vi "Ensure Channel.vi"(8 "error in (no error)":errorcluster, 10 "Name":string, 11 "SignalManager in":refnum<class "SignalManager.lvclass">) -> (0 "error out":errorcluster, 3 "SignalManager out":refnum<class "SignalManager.lvclass">)   [LabVIEW 2015, in "SignalManager.lvclass"]
uses:
  SignalManager.lvclass
  SignalManager.lvclass/SignalManager.ctl
  Channel/Channel.lvclass
  Channel/Channel.lvclass/Channel.ctl
  Channel/Write Name.vi
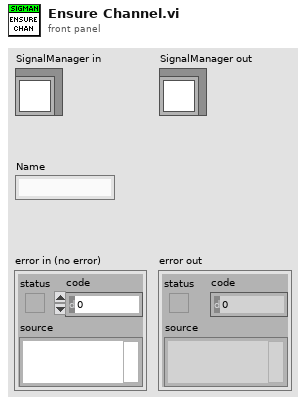
[diagram p1: front panel]
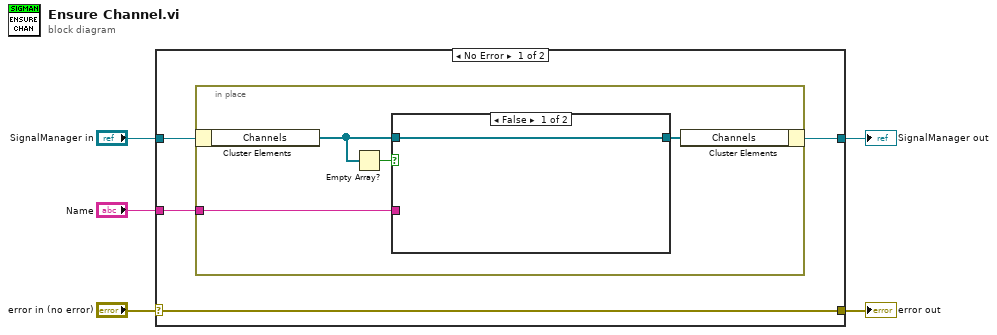
[diagram p0: block diagram]
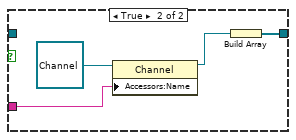
[diagram p2: hidden frame]
diagram:
  n1 = case shown="No Error" "error in (no error)" {
    selector: "error in (no error)" -> [w9 w20]
    tunnel: [w9 w20] -> w4
    tunnel: [w7 w19] -> w2
    tunnel: "SignalManager in" -> [w8 w19]
    tunnel: "Name" -> [w6 _]
    frame No Error {
      n2 = in-place {
        in-place-border: w6 -> [w10]
        n3 = in-place-cluster #1(w8) -> ("Channels"=w11:refnum<class "Channel.lvclass">[])
        n4 = Empty Array?(array=w11) -> (empty?=w12:bool)
        n5 = case shown="False" w12 {
          tunnel: [w14 w18] -> w13
          tunnel: w11 -> [w14 _]
          tunnel: w10 -> [_ w15]
          frame False {
          }
          frame True {
            n6 = property class="Channel"(reference=refnum<class "Channel.lvclass"> refnum ("Channel"), "Accessors:Name"=w15) -> (reference out=w16:refnum<class "Channel.lvclass">)  [unwired: 1 in, 1 out]
            n7 = Build Array(w16) -> (w18:refnum<class "Channel.lvclass">[])
          }
        }
        n8 = in-place-cluster #1("Channels"=w13) -> (w7:refnum<class "SignalManager.lvclass">)
      }
    }
    frame Error {
    }
  }
  "error out" <- w4
  "SignalManager out" <- w2
